vi "ini_object_parse_string_array.vi"(8 "error in":errorcluster, 11 "string in":string) -> (0 "error out":errorcluster, 3 "string array out":string[](array[string]))   [LabVIEW 2018]
uses:
  <vilib>/regexp/Match Regular Expression.xnode
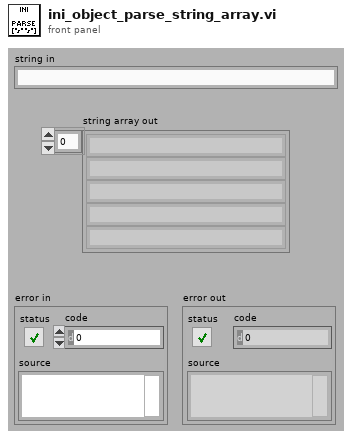
[diagram p1: front panel]
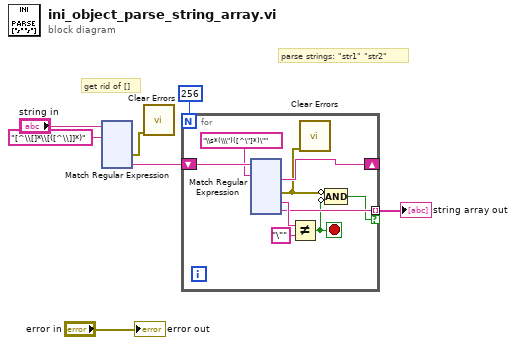
[diagram p0: block diagram]
diagram:
  # "parse strings: \"str1\" \"str2\""
  # "get rid of []"
  n1 = xnode "Match Regular Expression"("input string"="string in", "regular expression"="[^\\[]*\\[([^\\]]*)") -> ("error out"=w4:errorcluster, "submatch 1"=w3:string)  [unwired: 4 in, 4 out]
  n2 = call <vilib>:"Clear Errors.vi"("error in (no error)"=w4) -> ()  [unwired: 5 in, 2 out]
  n3 = for {
    N: 256 -> [_]
    tunnel: [w12] -> w2 mode=indexing if=w8
    shift-right: [w11] -> _
    shift-left: w3 -> [w16]
    stop <- w10 stop-if-true
    n4 = xnode "Match Regular Expression"("input string"=w16, "regular expression"="\\s*(\\\")([^\"]*)\"") -> ("after match"=w11:string, "error out"=w9:errorcluster, "submatch 1"=w14:string, "submatch 2"=w12:string)  [unwired: 4 in, 3 out]
    n5 = Not Equal?(x=w14, y="\"") -> (x != y?=w10:bool)
    n6 = call <vilib>:"Clear Errors.vi"("error in (no error)"=w9) -> ()  [unwired: 5 in, 2 out]
    n7 = Compound Arithmetic op=AND(invert w9, invert w10) -> (w8:bool)
  }
  "string array out" <- w2
  "error out" <- "error in"
